vi "HVBuncher.ProcCases.vi"(0 "i ref in":refnum<vi>, 1 "selector":string, 2 "Data":T1, 3 "call cluster":T2={"Object"="", "Selector"="", "CallType"=enum."synchronous", "Async Object"="", "Async Selector"="", "Data Descriptor"="", "Data"=[], "Error #"=0, "Expire"=0}, 5 "error in (no error)":errorcluster) -> (14 "i ref out":refnum<vi>, 17 "answer cluster":T2={"Object"="", "Selector"="", "CallType"=enum."synchronous", "Async Object"="", "Async Selector"="", "Data Descriptor"="", "Data"=[], "Error #"=0, "Expire"=0}, 19 "error out":errorcluster)   [LabVIEW 2014, in "HVBuncher.lvlib"]
doc: "This method is called by a process from within the default case in the event loop. The methods of a class that are linked to events will be called from THIS method. Add your code here."
uses:
  HVBuncher.lvlib
  CS_Core/CSSystem/CoreDefs/CoreDefs.call_type.ctl
  CS_Core/BaseProcess/BaseProcess.descriptor string definition.ctl
  CS_Core/CSSystem/CoreDefs/CoreDefs.rawDataType.ctl
  CS_Core/CSSystem/CoreLib/CoreLib.byte array 2 double.vi
  CS_Core/CSSystem/CoreLib/CoreLib.double 2 byte array.vi
  CS_Core/CSSystem/CoreLib/CoreLib.string 2 byte array.vi
  CS_Core/CSSystem/CoreLib/CoreLib.byte array 2 int.vi
  CS_Core/CSSystem/CoreLib/CoreLib.byte array 2 short.vi
  CS_Core/CSSystem/CoreLib/CoreLib.lvlib
  CS_Core/BaseProcess/BaseProcess.lvlib
  CS_Core/CSApplicationBaseClasses/PSChannelBase/PSChannelBase.lvlib
  CS_Core/CAEObj/CAEObj.lvlib
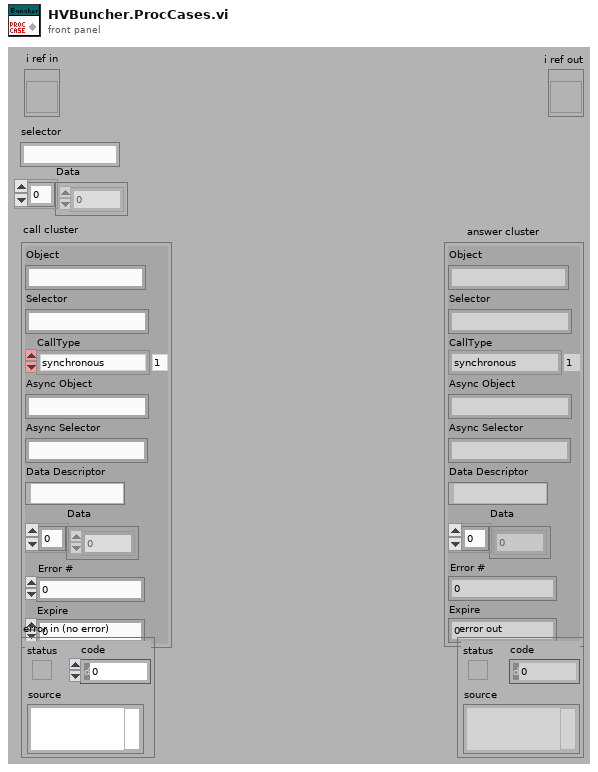
[diagram p1: front panel]
types:
  T1 = typedef "CoreDefs.rawDataType.ctl" = i8[]
  T2 = typedef "CoreDefs.call_type.ctl" = cluster{"Object":string, "Selector":string, "CallType":enum16{"simple", "synchronous", "asynchronous"}, "Async Object":string, "Async Selector":string, "Data Descriptor":T3, "Data":T1, "Error #":i32, "Expire":u32}
  T3 = typedef "BaseProcess.lvlib/BaseProcess.descriptor string definition.ctl" = string
  T4 = typedef "HVBuncher.lvlib/HVBuncher.i attribute.ctl" = cluster{"ObjectsInitialized":bool, "ChildObjects":T5}
  T5 = typedef "HVBuncher.lvlib/HVBuncher.ChildObjects.ctl" = cluster{"ObjectsLoaded":string[], "actVoltage":dbl[]}
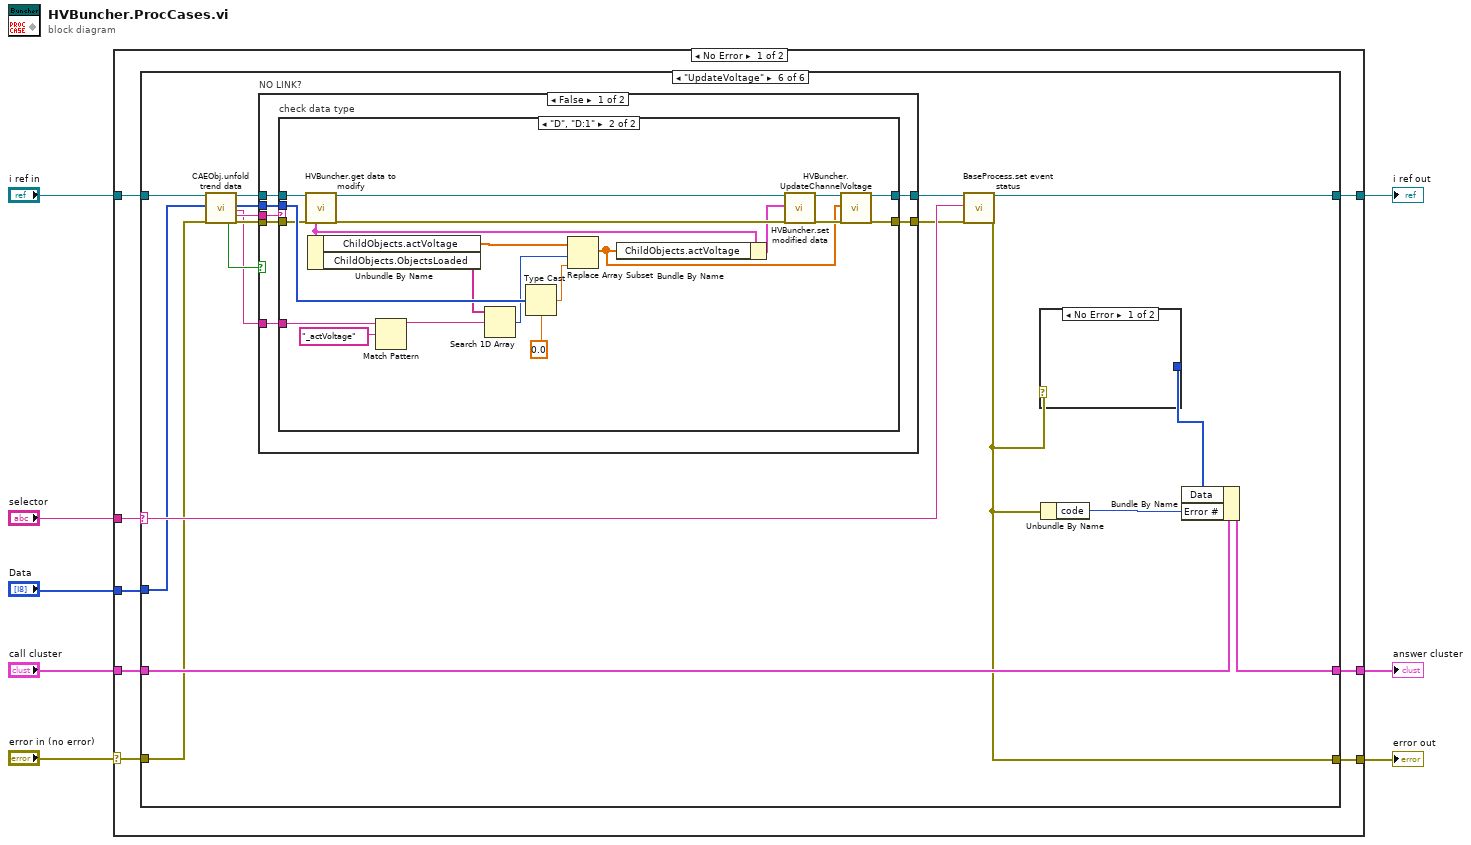
[diagram p0: block diagram]
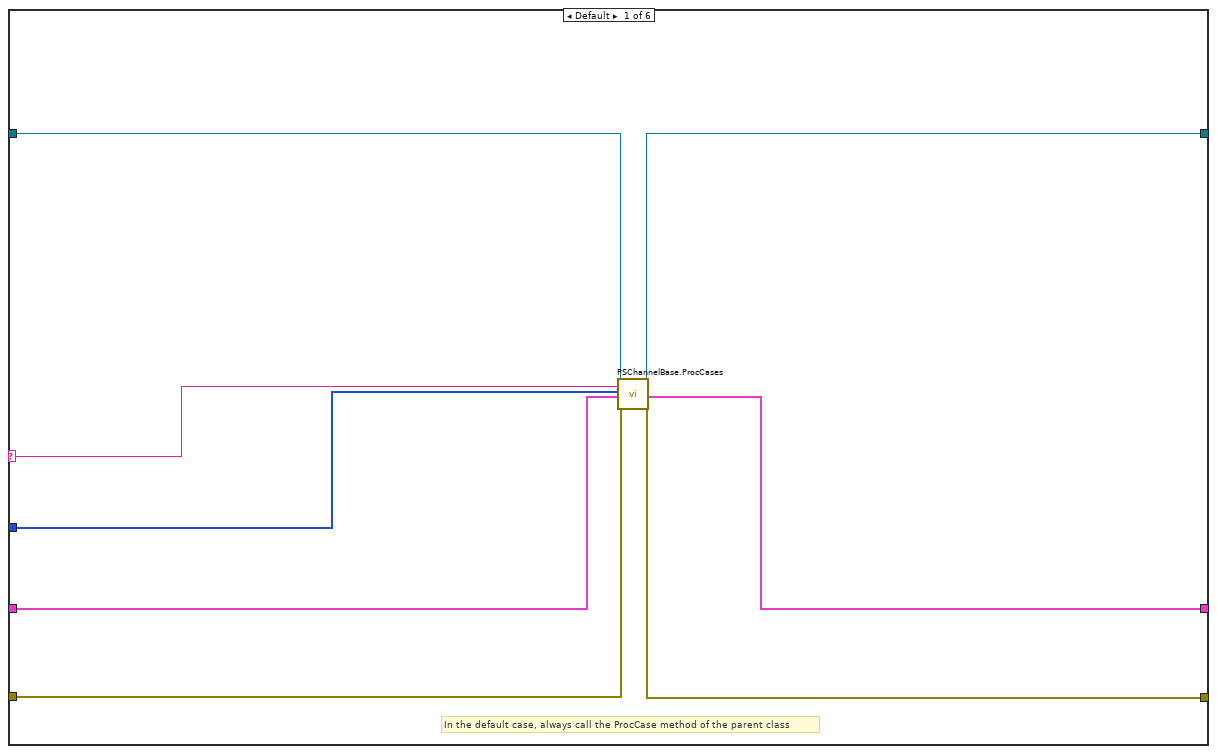
[diagram p2: hidden frame]
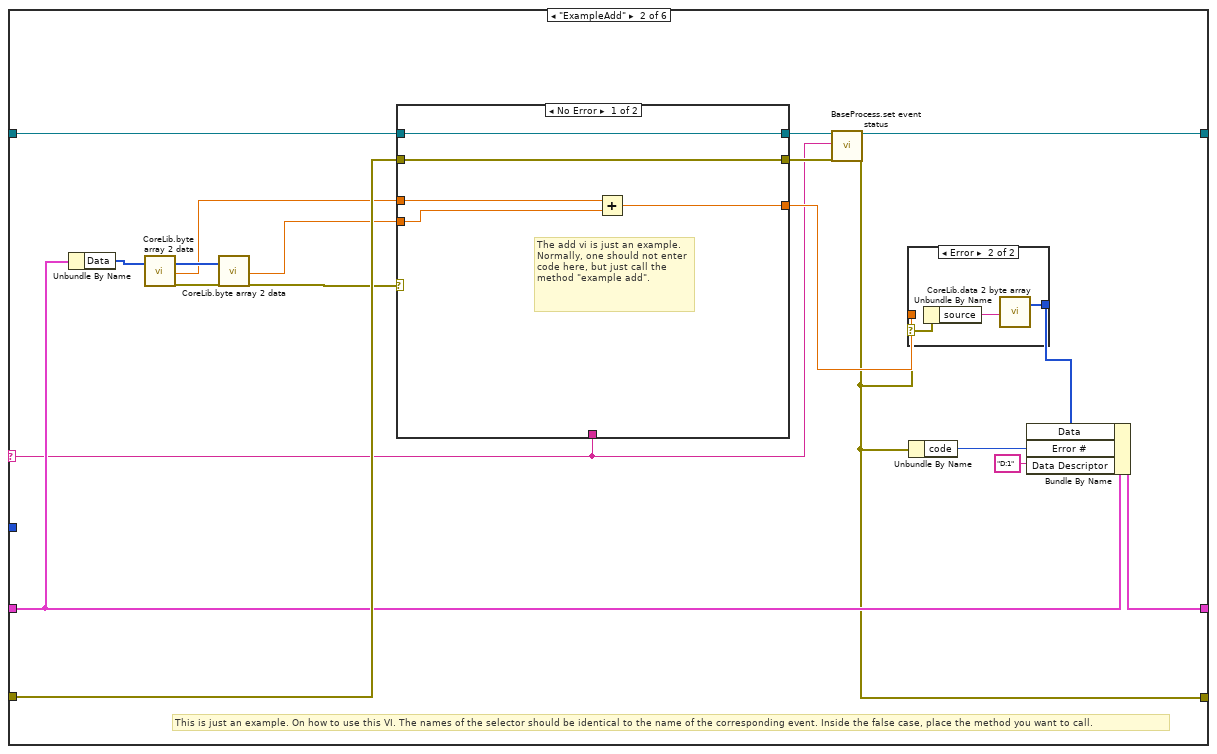
[diagram p3: hidden frame]
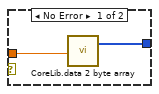
[diagram p4: hidden frame]
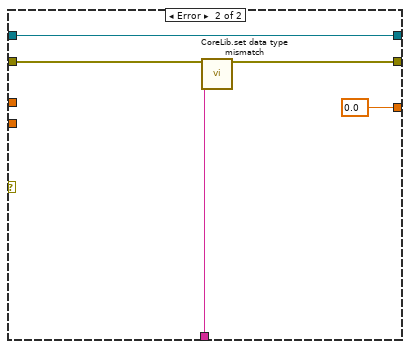
[diagram p5: hidden frame]
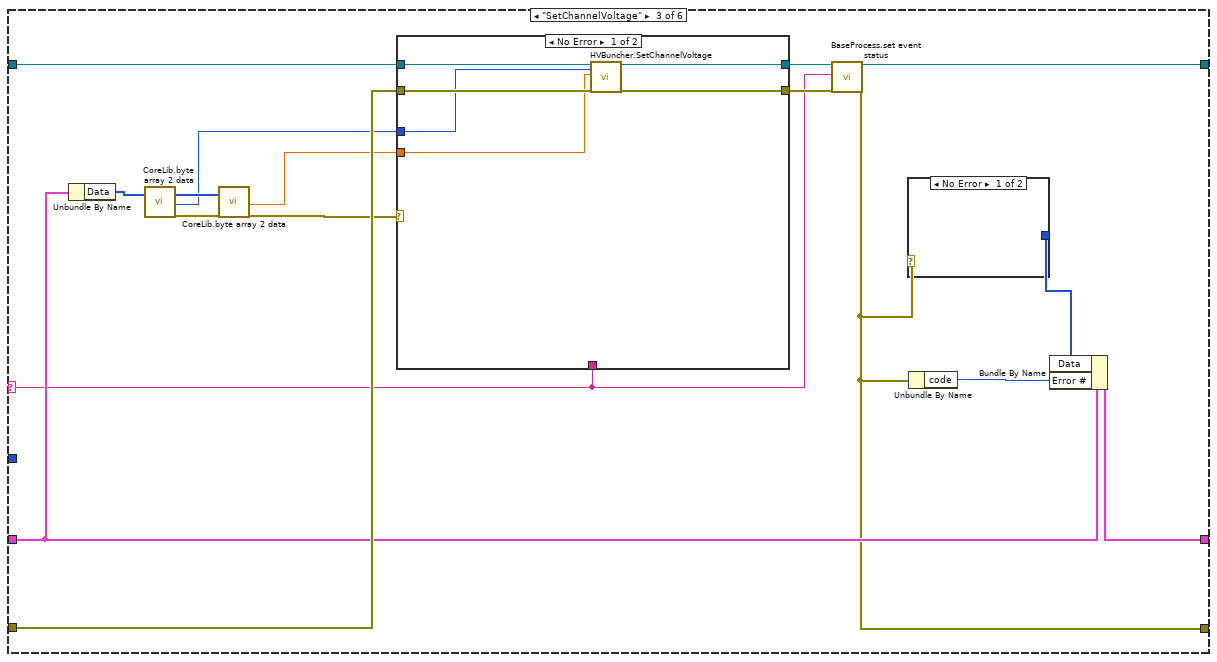
[diagram p6: hidden frame]
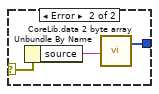
[diagram p7: hidden frame]
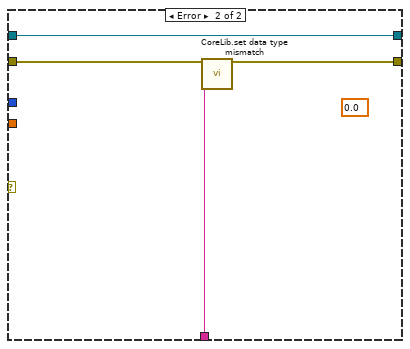
[diagram p8: hidden frame]
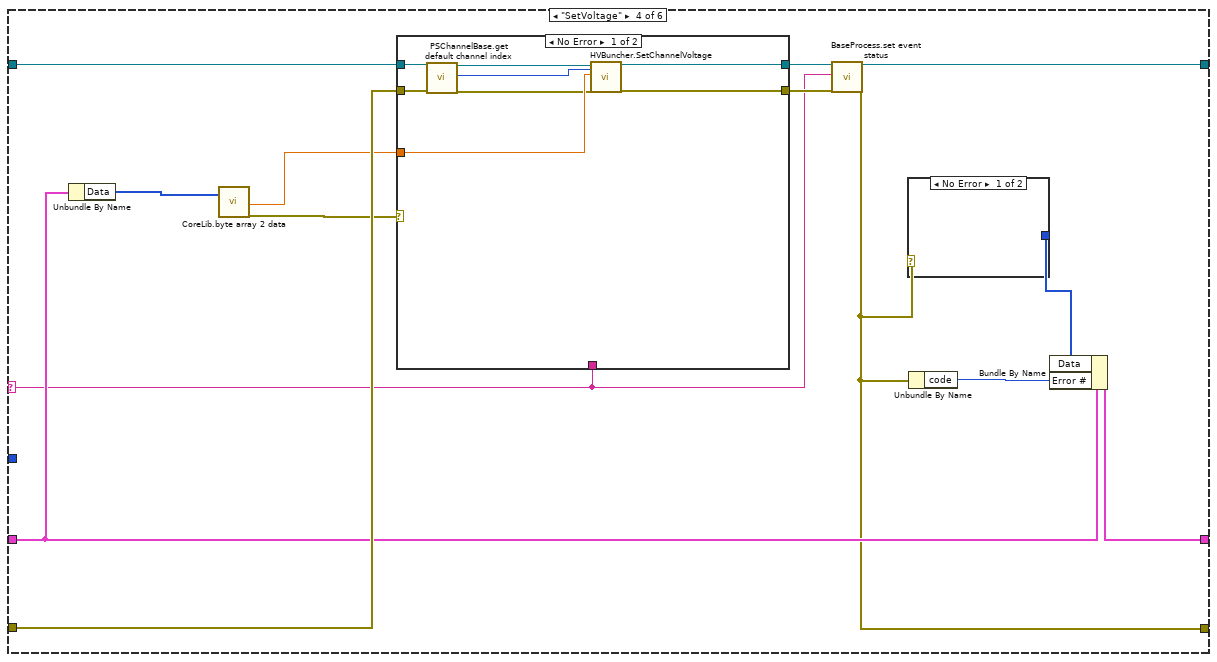
[diagram p9: hidden frame]
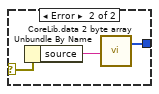
[diagram p10: hidden frame]
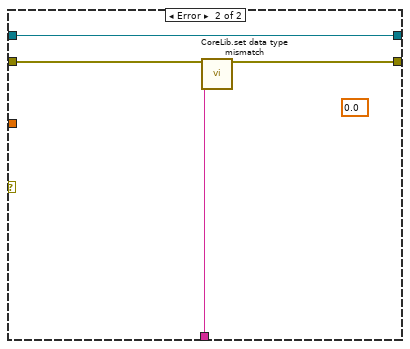
[diagram p11: hidden frame]
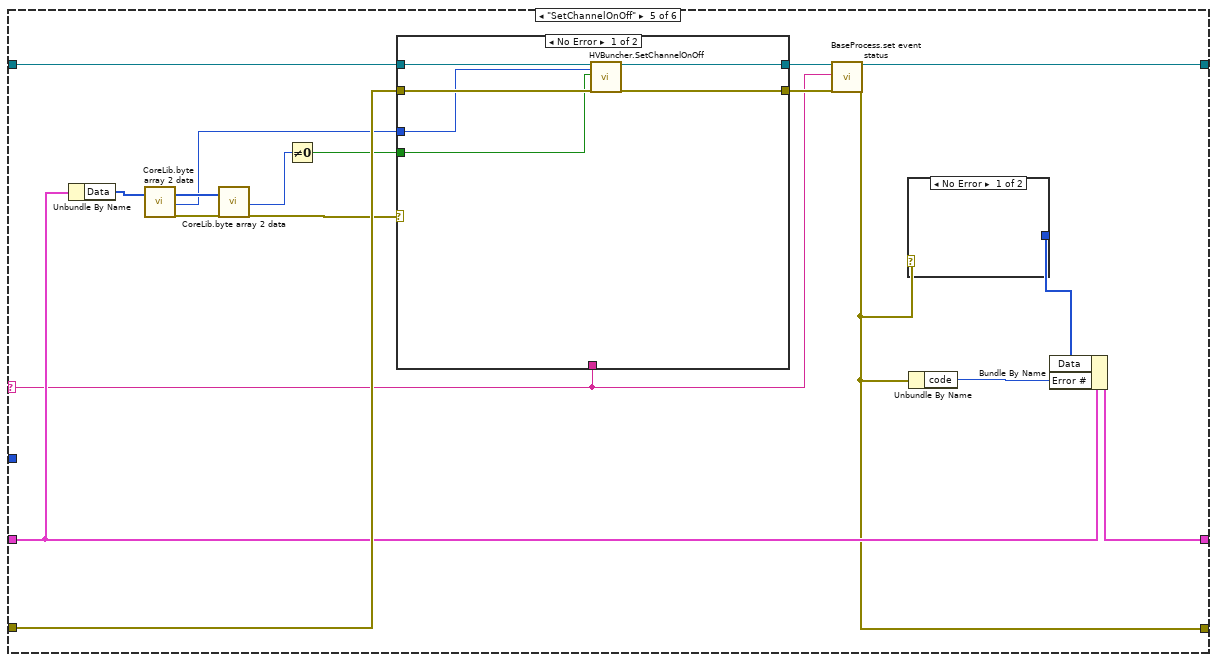
[diagram p12: hidden frame]
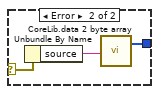
[diagram p13: hidden frame]
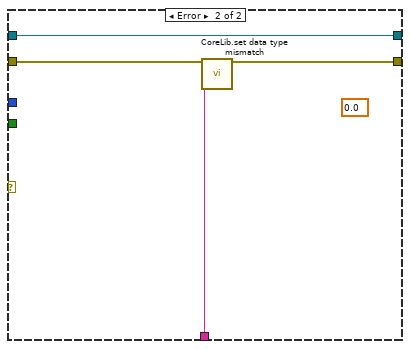
[diagram p14: hidden frame]
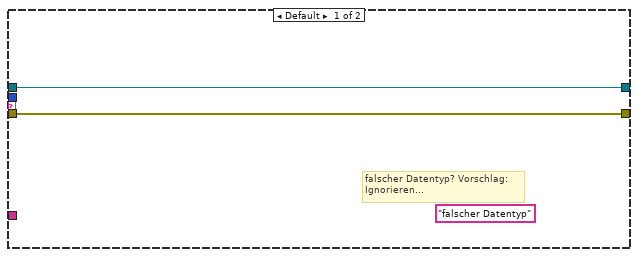
[diagram p15: hidden frame]
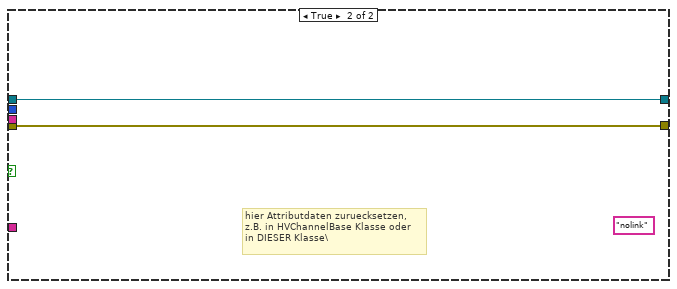
[diagram p16: hidden frame]
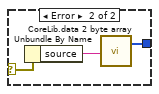
[diagram p17: hidden frame]
diagram:
  n1 = case shown="No Error" "error in (no error)" {
    selector: "error in (no error)" -> [w9 w201]
    tunnel: "selector" -> [w16 _]
    tunnel: [w15 w202] -> w7
    tunnel: "Data" -> [w14 _]
    tunnel: "call cluster" -> [w13 w202]
    tunnel: "i ref in" -> [w12 w203]
    tunnel: [w11 w203] -> w3
    tunnel: [w10 w201] -> w2
    frame No Error {
      n2 = case shown="\"UpdateVoltage\"" w16 {
        selector: w16 -> [w19 w33 w66 w93 w126 w161]
        tunnel: w14 -> [w17 _ _ _ _ w157]
        tunnel: w12 -> [w18 w43 w75 w102 w135 w159]
        tunnel: [w24 w32 w65 w92 w125 w160] -> w11
        tunnel: w13 -> [w20 w39 w72 w99 w132 w165]
        tunnel: [w21 w38 w71 w98 w131 w164] -> w15
        tunnel: w9 -> [w23 w42 w74 w101 w134 w158]
        tunnel: [w22 w34 w67 w94 w127 w162] -> w10
        frame Default {
          # "In the default case, always call the ProcCase method of the parent class"
          n3 = call "PSChannelBase.ProcCases.vi"("i ref in"=w18, "selector"=w19, "Data"=w17, "call cluster"=w20, "error in (no error)"=w23) -> ("i ref out"=w24:refnum<vi>, "answer cluster"=w21:T2, "error out"=w22:errorcluster)  [unwired: 12 in]
        }
        frame "ExampleAdd" {
          # "This is just an example. On how to use this VI. The names of the selector should be identical to the name of the corresponding event. Inside the false case, place the method you want to call."
          n4 = Unbundle By Name(w39) -> ("Data"=w30:T1)
          n5 = call-poly "CoreLib.byte array 2 data.vi"("byteArray"=w30) -> ("byteArray out"=w28:T1, "d64"=w26:dbl, "error out"=w29:errorcluster)  [unwired: 16 in]
          n6 = call-poly "CoreLib.byte array 2 data.vi"("byteArray"=w28, "error in (no error)"=w29) -> ("d64"=w25:dbl, "error out"=w27:errorcluster)  [unwired: 15 in, 1 out]
          n7 = case shown="No Error" w27 {
            tunnel: [w50 w58] -> w36
            tunnel: w43 -> [w50 w58]
            tunnel: w42 -> [w51 w57]
            tunnel: [w51 w56] -> w35
            tunnel: w25 -> [w53 _]
            tunnel: [w52 0.0] -> w41
            tunnel: w33 -> [_ w54]
            tunnel: w26 -> [w49 _]
            frame No Error {
              # "The add vi is just an example. Normally, one should not enter code here, but just call the method \"example add\"."
              n8 = Add(x=w49, y=w53) -> (x+y=w52:dbl)
            }
            frame Error {
              n9 = call "CoreLib.set data type mismatch.vi"("error in (no error)"=w57, "error source"=w54) -> ("error out"=w56:errorcluster)  [unwired: 17 in]
            }
          }
          n10 = call "BaseProcess.set event status.vi"("i ref in"=w36, "EventStatus"=w33, "error in (no error)"=w35) -> ("i ref out"=w32:refnum<vi>, "error out"=w34:errorcluster)  [unwired: 14 in, 1 out]
          n11 = case shown="Error" w34 {
            selector: w34 -> [_ w48]
            tunnel: [w44 w47] -> w37
            tunnel: w41 -> [w45 _]
            frame No Error {
              n12 = call-poly "CoreLib.data 2 byte array.vi"("f64"=w45) -> ("byteArray out"=w44:T1)  [unwired: 18 in]
            }
            frame Error {
              n13 = Unbundle By Name(w48) -> ("source"=w46:string)
              n14 = call-poly "CoreLib.data 2 byte array.vi"("string"=w46) -> ("byteArray out"=w47:T1)  [unwired: 18 in]
            }
          }
          n15 = Unbundle By Name(w34) -> ("code"=w40:i32)
          n16 = Bundle By Name(cluster=w39, "Data"=w37, "Error #"=w40, "Data Descriptor"="D:1") -> (w38:T2)
        }
        frame "SetChannelVoltage" {
          n17 = Unbundle By Name(w72) -> ("Data"=w64:T1)
          n18 = call-poly "CoreLib.byte array 2 data.vi"("byteArray"=w64) -> ("byteArray out"=w62:T1, "i32"=w60:i32, "error out"=w63:errorcluster)  [unwired: 16 in]
          n19 = call-poly "CoreLib.byte array 2 data.vi"("byteArray"=w62, "error in (no error)"=w63) -> ("d64"=w59:dbl, "error out"=w61:errorcluster)  [unwired: 15 in, 1 out]
          n20 = case shown="No Error" w61 {
            tunnel: [w83 w88] -> w69
            tunnel: w75 -> [w84 w88]
            tunnel: w74 -> [w81 w87]
            tunnel: [w82 w86] -> w68
            tunnel: w59 -> [w79 _]
            tunnel: w66 -> [_ w85]
            tunnel: w60 -> [w80 _]
            frame No Error {
              n21 = call "HVBuncher.SetChannelVoltage.vi"("i ref in"=w84, "channel"=w80, "Voltage in V"=w79, "error in (no error)"=w81) -> ("i ref out"=w83:refnum<vi>, "error out"=w82:errorcluster)  [unwired: 13 in, 1 out]
            }
            frame Error {
              (unwired) 0.0
              n22 = call "CoreLib.set data type mismatch.vi"("error in (no error)"=w87, "error source"=w85) -> ("error out"=w86:errorcluster)  [unwired: 17 in]
            }
          }
          n23 = call "BaseProcess.set event status.vi"("i ref in"=w69, "EventStatus"=w66, "error in (no error)"=w68) -> ("i ref out"=w65:refnum<vi>, "error out"=w67:errorcluster)  [unwired: 14 in, 1 out]
          n24 = case shown="No Error" w67 {
            selector: w67 -> [_ w78]
            tunnel: [_ w77] -> w70
            frame No Error {
            }
            frame Error {
              n25 = Unbundle By Name(w78) -> ("source"=w76:string)
              n26 = call-poly "CoreLib.data 2 byte array.vi"("string"=w76) -> ("byteArray out"=w77:T1)  [unwired: 18 in]
            }
          }
          n27 = Unbundle By Name(w67) -> ("code"=w73:i32)
          n28 = Bundle By Name(cluster=w72, "Data"=w70, "Error #"=w73) -> (w71:T2)
        }
        frame "SetVoltage" {
          n29 = Unbundle By Name(w99) -> ("Data"=w89:T1)
          n30 = call-poly "CoreLib.byte array 2 data.vi"("byteArray"=w89) -> ("d64"=w90:dbl, "error out"=w91:errorcluster)  [unwired: 16 in, 1 out]
          n31 = case shown="No Error" w91 {
            tunnel: [w113 w117] -> w96
            tunnel: w102 -> [w110 w117]
            tunnel: w101 -> [w109 w116]
            tunnel: [w112 w115] -> w95
            tunnel: w90 -> [w111 _]
            tunnel: w93 -> [_ w114]
            frame No Error {
              n32 = call "PSChannelBase.get default channel index.vi"("i ref in"=w110, "error in (no error)"=w109) -> ("i ref out"=w107:refnum<vi>, "defaultChannelIndex"=w106:i32, "error out"=w108:errorcluster)  [unwired: 15 in]
              n33 = call "HVBuncher.SetChannelVoltage.vi"("i ref in"=w107, "channel"=w106, "Voltage in V"=w111, "error in (no error)"=w108) -> ("i ref out"=w113:refnum<vi>, "error out"=w112:errorcluster)  [unwired: 13 in, 1 out]
            }
            frame Error {
              (unwired) 0.0
              n34 = call "CoreLib.set data type mismatch.vi"("error in (no error)"=w116, "error source"=w114) -> ("error out"=w115:errorcluster)  [unwired: 17 in]
            }
          }
          n35 = call "BaseProcess.set event status.vi"("i ref in"=w96, "EventStatus"=w93, "error in (no error)"=w95) -> ("i ref out"=w92:refnum<vi>, "error out"=w94:errorcluster)  [unwired: 14 in, 1 out]
          n36 = case shown="No Error" w94 {
            selector: w94 -> [_ w105]
            tunnel: [_ w104] -> w97
            frame No Error {
            }
            frame Error {
              n37 = Unbundle By Name(w105) -> ("source"=w103:string)
              n38 = call-poly "CoreLib.data 2 byte array.vi"("string"=w103) -> ("byteArray out"=w104:T1)  [unwired: 18 in]
            }
          }
          n39 = Unbundle By Name(w94) -> ("code"=w100:i32)
          n40 = Bundle By Name(cluster=w99, "Data"=w97, "Error #"=w100) -> (w98:T2)
        }
        frame "SetChannelOnOff" {
          n41 = Unbundle By Name(w132) -> ("Data"=w124:T1)
          n42 = call-poly "CoreLib.byte array 2 data.vi"("byteArray"=w124) -> ("byteArray out"=w122:T1, "i32"=w120:i32, "error out"=w123:errorcluster)  [unwired: 16 in]
          n43 = call-poly "CoreLib.byte array 2 data.vi"("byteArray"=w122, "error in (no error)"=w123) -> ("i16"=w119:i16, "error out"=w121:errorcluster)  [unwired: 15 in, 1 out]
          n44 = Not Equal To 0?(x=w119) -> (x != 0?=w118:bool)
          n45 = case shown="No Error" w121 {
            tunnel: [w143 w148] -> w129
            tunnel: w135 -> [w144 w148]
            tunnel: w134 -> [w141 w147]
            tunnel: [w142 w146] -> w128
            tunnel: w118 -> [w139 _]
            tunnel: w126 -> [_ w145]
            tunnel: w120 -> [w140 _]
            frame No Error {
              n46 = call "HVBuncher.SetChannelOnOff.vi"("i ref in"=w144, "ChannelNr"=w140, "SetOnOff"=w139, "error in (no error)"=w141) -> ("i ref out"=w143:refnum<vi>, "error out"=w142:errorcluster)  [unwired: 13 in, 1 out]
            }
            frame Error {
              (unwired) 0.0
              n47 = call "CoreLib.set data type mismatch.vi"("error in (no error)"=w147, "error source"=w145) -> ("error out"=w146:errorcluster)  [unwired: 17 in]
            }
          }
          n48 = call "BaseProcess.set event status.vi"("i ref in"=w129, "EventStatus"=w126, "error in (no error)"=w128) -> ("i ref out"=w125:refnum<vi>, "error out"=w127:errorcluster)  [unwired: 14 in, 1 out]
          n49 = case shown="No Error" w127 {
            selector: w127 -> [_ w138]
            tunnel: [_ w137] -> w130
            frame No Error {
            }
            frame Error {
              n50 = Unbundle By Name(w138) -> ("source"=w136:string)
              n51 = call-poly "CoreLib.data 2 byte array.vi"("string"=w136) -> ("byteArray out"=w137:T1)  [unwired: 18 in]
            }
          }
          n52 = Unbundle By Name(w127) -> ("code"=w133:i32)
          n53 = Bundle By Name(cluster=w132, "Data"=w130, "Error #"=w133) -> (w131:T2)
        }
        frame "UpdateVoltage" {
          n54 = call "CAEObj.unfold trend data.vi"("i ref in"=w159, "raw trend data"=w157, "error in (no error)"=w158) -> ("no link"=w156:bool, "i ref out"=w155:refnum<vi>, "data"=w150:i8[], "serviceName"=w149:string, "typeDescriptor"=w151:string, "error out"=w154:errorcluster)  [unwired: 8 in, 3 out]
          n55 = case "NO LINK?" shown="False" w156 {
            tunnel: w155 -> [w172 w197]
            tunnel: w154 -> [w170 w196]
            tunnel: [w171 w197] -> w153
            tunnel: [w169 w196] -> w152
            tunnel: w151 -> [w173 _]
            tunnel: w150 -> [w168 _]
            tunnel: w149 -> [w167 _]
            frame False {
              n56 = case "check data type" shown="\"D\", \"D:1\"" w173 {
                tunnel: w172 -> [w175 w190]
                tunnel: [w175 w180] -> w171
                tunnel: w170 -> [w174 w189]
                tunnel: [w174 w179] -> w169
                tunnel: w168 -> [_ w195]
                tunnel: w167 -> [_ w194]
                frame Default {
                  (unwired) "falscher Datentyp"
                  # "falscher Datentyp? Vorschlag: \nIgnorieren..."
                }
                frame "D", "D:1" {
                  n57 = call "HVBuncher.get data to modify.vi"("i ref in"=w190, "error in (no error)"=w189) -> ("i ref out"=w187:refnum<vi>, "i attribute"=w182:T4, "error out"=w186:errorcluster)  [unwired: 14 in, 1 out]
                  n58 = Unbundle By Name(w182) -> ("ChildObjects.actVoltage"=w184:dbl[], "ChildObjects.ObjectsLoaded"=w188:string[])
                  n59 = Match Pattern(string=w194, regular expression="_actVoltage") -> (before substring=w191:string)  [unwired: 1 in, 3 out]
                  n60 = Search 1D Array(1D array=w188, element=w191) -> (index of element=w181:i32)  [unwired: 1 in]
                  n61 = Type Cast(type=0.0, x=w195) -> (*(type *) &x=w185:dbl)
                  n62 = Replace Array Subset(array=w184, new element=w185, index=w181) -> (w176:dbl[])
                  n63 = Bundle By Name(cluster=w182, "ChildObjects.actVoltage"=w176) -> (w183:T4)
                  n64 = call "HVBuncher.set modified data.vi"("i ref in"=w187, "i attribute"=w183, "error in (no error)"=w186) -> ("i ref out"=w178:refnum<vi>, "error out"=w177:errorcluster)  [unwired: 15 in]
                  n65 = call "HVBuncher.UpdateChannelVoltage.vi"("i ref in"=w178, "ChannelVoltages"=w176, "error in (no error)"=w177) -> ("i ref out"=w180:refnum<vi>, "error out"=w179:errorcluster)  [unwired: 13 in, 2 out]
                }
              }
            }
            frame True {
              (unwired) "nolink"
              # "hier Attributdaten zuruecksetzen,\nz.B. in HVChannelBase Klasse oder\nin DIESER Klasse\\"
            }
          }
          n66 = call "BaseProcess.set event status.vi"("i ref in"=w153, "EventStatus"=w161, "error in (no error)"=w152) -> ("i ref out"=w160:refnum<vi>, "error out"=w162:errorcluster)  [unwired: 14 in, 1 out]
          n67 = case shown="No Error" w162 {
            selector: w162 -> [_ w200]
            tunnel: [_ w199] -> w163
            frame No Error {
            }
            frame Error {
              n68 = Unbundle By Name(w200) -> ("source"=w198:string)
              n69 = call-poly "CoreLib.data 2 byte array.vi"("string"=w198) -> ("byteArray out"=w199:T1)  [unwired: 18 in]
            }
          }
          n70 = Unbundle By Name(w162) -> ("code"=w166:i32)
          n71 = Bundle By Name(cluster=w165, "Data"=w163, "Error #"=w166) -> (w164:T2)
        }
      }
    }
    frame Error {
    }
  }
  "answer cluster" <- w7
  "i ref out" <- w3
  "error out" <- w2
